vi "read_master_file.vi"(8 "error in (no error)":errorcluster, 10 "setup file pattern":string[](array[string]), 11 "master file path":path) -> (0 "error out":errorcluster, 3 "setup file paths":string)   [LabVIEW 2017, in "worker.lvlib"]
uses:
  worker.lvlib
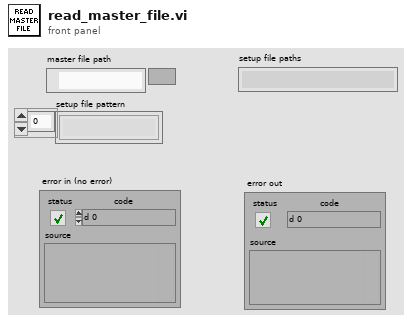
[diagram p1: front panel]
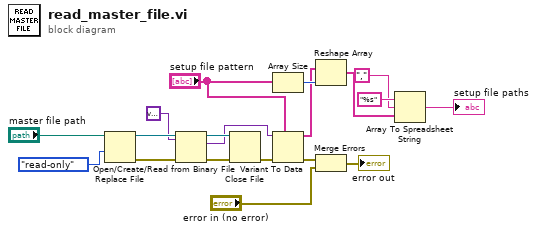
[diagram p0: block diagram]
diagram:
  n1 = Open/Create/Replace File(file path (use dialog)="master file path", access (0:read/write)=enum16{"read/write", "read-only", "write-only"}."read-only") -> (refnum out=w17:refnum<file>, error out=w18:errorcluster)  [unwired: 4 in, 1 out]
  n2 = Read from Binary File(5:variant, 8:w18, 11:w17) -> (0:w15:errorcluster, 2:w13:variant, 3:w14:refnum<file>)  [unwired: 3 in, 1 out]
  n3 = Close File(refnum=w14, error in=w15) -> (error out=w9:errorcluster)  [unwired: 1 out]
  n4 = Array Size(array="setup file pattern") -> (size(s)=w12:i32)
  n5 = Variant To Data(error in=w9, type="setup file pattern", Variant=w13) -> (data=w2:string[], error out=w6:errorcluster)
  n6 = Reshape Array(w2, w12) -> (w3:string[])
  n7 = Merge Errors(w6, "error in (no error)") -> (→"error out":errorcluster)
  n8 = Array To Spreadsheet String(delimiter (Tab)=",", array=w3, 3:"%s" ("format string")) -> (spreadsheet string=→"setup file paths":string)
